vi "Parse HTTP Response.vi"(8 "error in (no error)":errorcluster, 11 "HTTP Response":string) -> (0 "error out":errorcluster, 2 "Body":string, 3 "Header":string)   [LabVIEW 2017, in "Feed.lvclass"]
uses:
  <vilib>/NI_RSS/Feed/Feed.lvclass
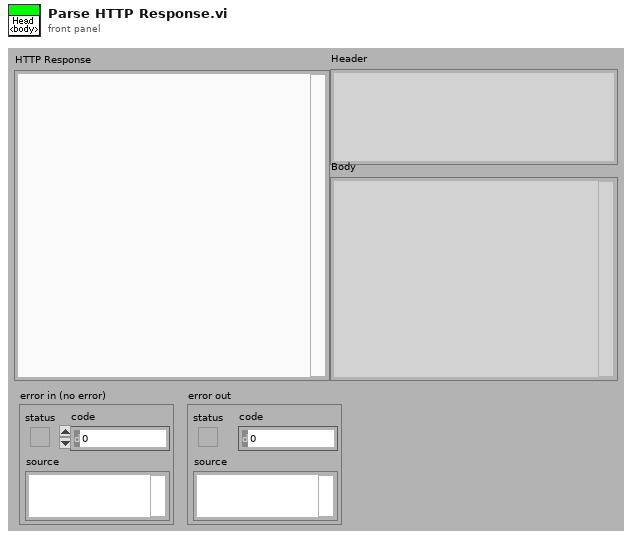
[diagram p1: front panel]
types:
  T1 = enum16{"Native", "Native Command Line", "UNIX", "Macintosh", "DOS"}
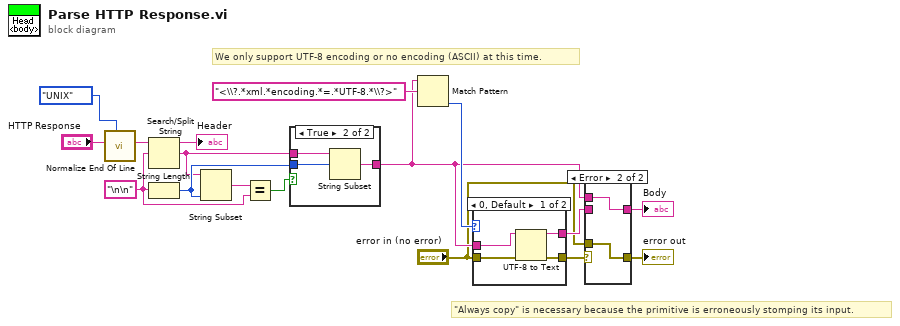
[diagram p0: block diagram]
diagram:
  w13 = "\n\n" ("regular expression")
  # "\"Always copy\" is necessary because the primitive is erroneously stomping its input."
  # "We only support UTF-8 encoding or no encoding (ASCII) at this time."
  n1 = call <vilib>:"Normalize End Of Line.vi"("end of line (Native)"=T1."UNIX" ("End Of Line (Native)"), "string in"="HTTP Response") -> ("string out"=w15:string)  [unwired: 6 out]
  n2 = Search/Split String(string=w15, search string/char (-)=w13) -> (substring before match=→"Header":string, match + rest of string=w10:string)  [unwired: 1 in, 1 out]
  n3 = String Length(string=w13) -> (length=w11:i32)
  n4 = String Subset(string=w10, length (rest)=w11) -> (substring=w14:string)  [unwired: 1 in]
  n5 = Equal?(x=w14, y=w13) -> (x = y?=w12:bool)
  n6 = case shown="True" w12 {
    tunnel: w10 -> [w18 w21]
    tunnel: w11 -> [_ w20]
    tunnel: [w18 w19] -> w2
    frame False {
    }
    frame True {
      n7 = String Subset(string=w21, offset (0)=w20) -> (substring=w19:string)  [unwired: 1 in]
    }
  }
  n8 = Match Pattern(string=w2, regular expression="<\\?.*xml.*encoding.*=.*UTF-8.*\\?>") -> (offset past match=w7:i32)  [unwired: 1 in, 3 out]
  n9 = case shown="0, Default" w7 {
    tunnel: w2 -> [w25 w27]
    tunnel: [w24 w27] -> w5
    tunnel: "error in (no error)" -> [w22 w26]
    tunnel: [w23 w26] -> w6
    frame 0, Default {
      n10 = UTF-8 to Text(8:w22, 11:w25) -> (0:w23:errorcluster, 3:w24:string)  [unwired: 1 in]
    }
    frame -1 {
    }
  }
  n11 = case shown="Error" w6 {
    selector: w6 -> [w28 _]
    tunnel: [w29 w31] -> w4
    tunnel: w5 -> [w29 _]
    tunnel: [w28 w30] -> w3
    tunnel: w2 -> [_ w31]
    tunnel: "error in (no error)" -> [_ w30]
    frame No Error {
    }
    frame Error {
    }
  }
  "Body" <- w4
  "error out" <- w3
